vi "MattesImageRegistration.vi"(6 "Epsilon":dbl=0.01, 8 "error in (no error)":errorcluster, 9 "Starting Radius":dbl=10.0, 10 "Moving image in":T1=refnum, 11 "Fixed image in":T1=refnum) -> (0 "error out":errorcluster, 1 "False color alignment image":T1, 2 "Moving image out (duplicate)":T1, 3 "Fixed image out (duplicate)":T1, 4 "alignment quality":dbl=-0.39635115330155946, 5 "y translation":dbl=4.5810062720041405, 7 "x translation":dbl=-23.66339978067731)   [LabVIEW 2012]
uses:
  <vilib>/vision/Image Controls.llb/IMAQ Image.ctl
  <vilib>/vision/NI_Vision_Development_Module.lvlib
  C++/bin/Release/ImageReg.dll
panel:
  in  "maximum iteration":i32=200
  out "elapsed time (ms)":u32=741
  in  "Sampling Percentage":dbl=0.2
  out "# of iterations":dbl=100.0
  out "False color image":T1(plugin-control)
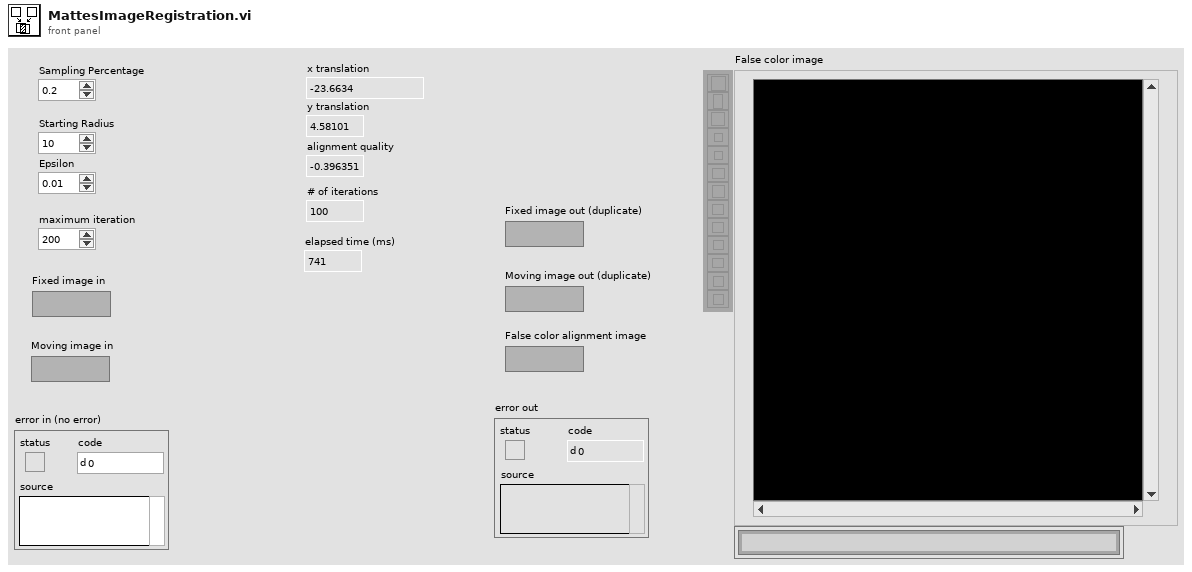
[diagram p1: front panel]
types:
  T1 = typedef "IMAQ Image.ctl" = refnum<image>
  T2 = typedef "Image Type" = u32
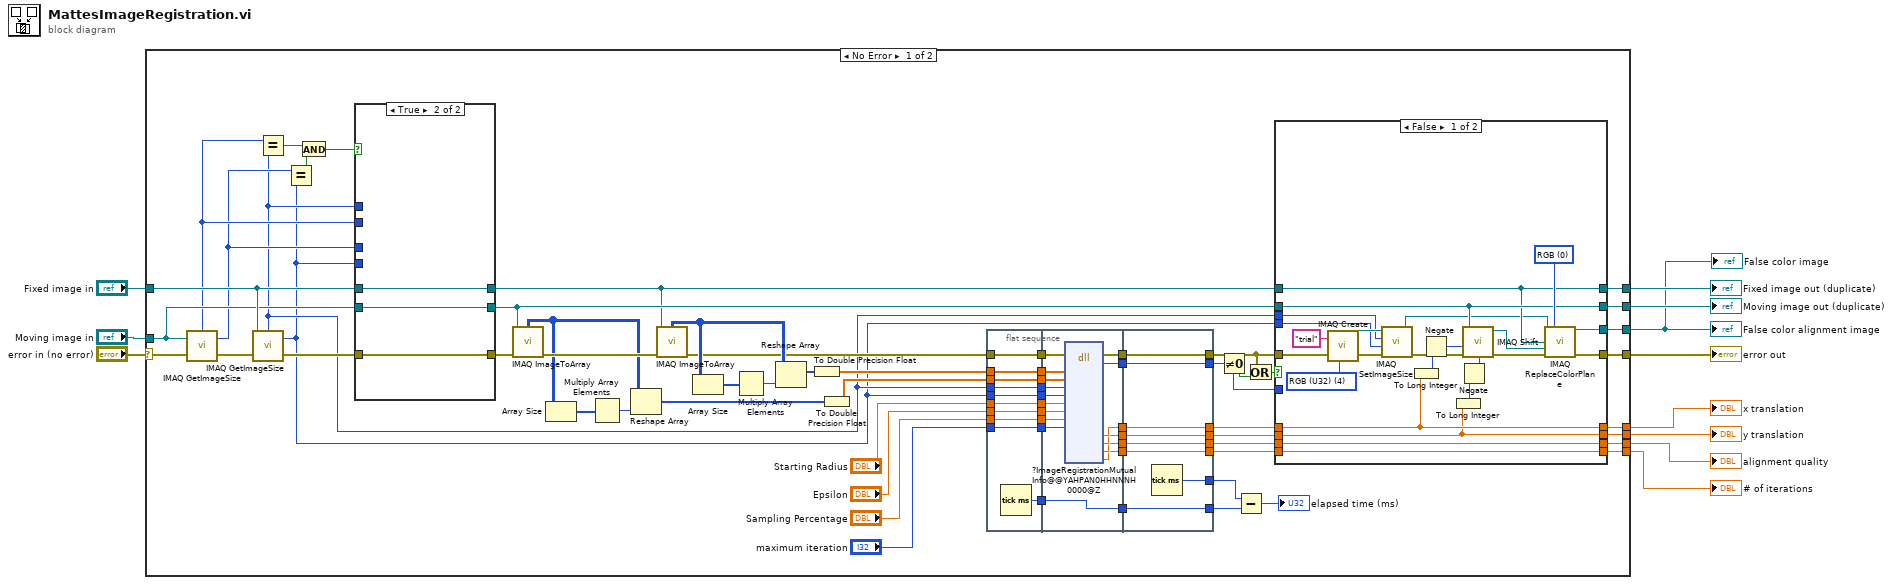
[diagram p0: block diagram]
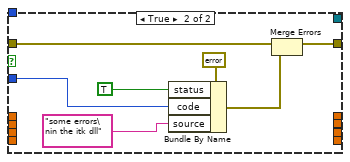
[diagram p2: hidden frame]
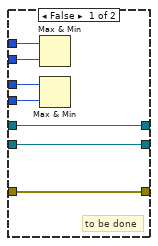
[diagram p3: hidden frame]
diagram:
  n1 = case shown="No Error" "error in (no error)" {
    selector: "error in (no error)" -> [w78 w154]
    tunnel: [w62 w154] -> w10
    tunnel: "Moving image in" -> [w72 _]
    tunnel: "Fixed image in" -> [w73 _]
    tunnel: [w53 _] -> w7
    tunnel: [w52 _] -> w6
    tunnel: [w51 _] -> w5
    tunnel: [w50 _] -> w2
    tunnel: [w49 _] -> w4
    tunnel: [w48 _] -> w3
    tunnel: [w47 _] -> w1
    frame No Error {
      n2 = call "IMAQ GetImageSize"("Image"=w72, "error in (no error)"=w78) -> ("Y Resolution"=w70:i32, "X Resolution"=w71:i32, "error out"=w77:errorcluster)  [unwired: 2 in]
      n3 = call "IMAQ GetImageSize"("Image"=w73, "error in (no error)"=w77) -> ("Y Resolution"=w41:i32, "X Resolution"=w42:i32, "error out"=w69:errorcluster)  [unwired: 2 in]
      n4 = Equal?(x=w71, y=w42) -> (x = y?=w75:bool)
      n5 = Equal?(x=w70, y=w41) -> (x = y?=w76:bool)
      n6 = And(x=w75, y=w76) -> (x .and. y?=w74:bool)
      n7 = case shown="True" w74 {
        tunnel: [w146 w153] -> w54
        tunnel: w73 -> [w146 w153]
        tunnel: [w145 w152] -> w61
        tunnel: w72 -> [w145 w152]
        tunnel: w42 -> [w150 _]
        tunnel: w71 -> [w149 _]
        tunnel: w70 -> [w148 _]
        tunnel: w41 -> [w147 _]
        tunnel: [w144 w151] -> w67
        tunnel: w69 -> [w144 w151]
        frame False {
          # "to be done"
          n8 = Max & Min(x=w150, y=w149) -> ()  [unwired: 2 out]
          n9 = Max & Min(x=w148, y=w147) -> ()  [unwired: 2 out]
        }
        frame True {
        }
      }
      n10 = call "IMAQ ImageToArray"("error in (no error)"=w67, "Image"=w61) -> ("error out"=w68:errorcluster, "Image Pixels (U8)"=w60:u8[][])  [unwired: 2 in, 3 out]
      n11 = Array Size(array=w60) -> (size(s)=w59:i32[])
      n12 = Multiply Array Elements(1:w59) -> (0:w58:i32)
      n13 = Reshape Array(w60, w58) -> (w65:u8[])
      n14 = call "IMAQ ImageToArray"("error in (no error)"=w68, "Image"=w54) -> ("error out"=w46:errorcluster, "Image Pixels (U8)"=w55:u8[][])  [unwired: 2 in, 3 out]
      n15 = Array Size(array=w55) -> (size(s)=w57:i32[])
      n16 = Multiply Array Elements(1:w57) -> (0:w56:i32)
      n17 = Reshape Array(w55, w56) -> (w66:u8[])
      n18 = To Double Precision Float(number=w66) -> (double precision float=w44:dbl[])
      n19 = To Double Precision Float(number=w65) -> (double precision float=w43:dbl[])
      n20 = flat-sequence {
        tunnel: "Sampling Percentage" -> [w81]
        tunnel: "Epsilon" -> [w82]
        tunnel: "Starting Radius" -> [w83]
        tunnel: w41 -> [w84]
        tunnel: w42 -> [w85]
        tunnel: w43 -> [w86]
        tunnel: w44 -> [w87]
        tunnel: w46 -> [w88]
        tunnel: [w88] -> w32
        tunnel: [w87] -> w31
        tunnel: [w86] -> w30
        tunnel: [w85] -> w29
        tunnel: [w84] -> w28
        tunnel: [w83] -> w27
        tunnel: [w82] -> w26
        tunnel: [w81] -> w25
        tunnel: [w80] -> w17
        tunnel: [w79] -> w13
        tunnel: "maximum iteration" -> [w79]
        tunnel: w32 -> [w104]
        tunnel: w31 -> [w102]
        tunnel: w30 -> [w101]
        tunnel: w29 -> [w100]
        tunnel: w28 -> [w99]
        tunnel: w27 -> [w98]
        tunnel: w26 -> [w97]
        tunnel: w25 -> [w96]
        tunnel: [w103] -> w24
        tunnel: [w95] -> w23
        tunnel: [w94] -> w22
        tunnel: [w93] -> w21
        tunnel: [w92] -> w20
        tunnel: [w91] -> w19
        tunnel: w17 -> [w90]
        tunnel: [w90] -> w16
        tunnel: w13 -> [w89]
        tunnel: [w107] -> w33
        tunnel: [w108] -> w34
        tunnel: [w109] -> w35
        tunnel: [w110] -> w36
        tunnel: [w111] -> w37
        tunnel: [w112] -> w45
        tunnel: w24 -> [w112]
        tunnel: w23 -> [w111]
        tunnel: w22 -> [w110]
        tunnel: w21 -> [w109]
        tunnel: w20 -> [w108]
        tunnel: w19 -> [w107]
        tunnel: [w106] -> w18
        tunnel: w16 -> [w105]
        tunnel: [w105] -> w15
        frame #0 {
          n21 = Tick Count (ms)() -> (millisecond timer value=w80:u32)
        }
        frame #1 {
          n22 = dll-call lib="D:/Moroder/dependencies/ImageReg/C++/bin/Release/ImageReg.dll" fn="?ImageRegistrationMutualInfo@@YAHPAN0HHNNNH0000@Z"(error in=w104, "fixed image"=w102, "moving image"=w101, "image width"=w100, "image height"=w99, "starting radius"=w98, "epsilon"=w97, "sampling percentage"=w96, "maximum iteration"=w89) -> (error out=w103:errorcluster, "error flag"=w91:i32, "x translation"=w95:dbl, "y translation"=w94:dbl, "quality"=w93:dbl, "number of iterations"=w92:dbl)  [unwired: 14 in, 1 out]
        }
        frame #2 {
          n23 = Tick Count (ms)() -> (millisecond timer value=w106:u32)
        }
      }
      n24 = Not Equal To 0?(x=w33) -> (x != 0?=w64:bool)
      n25 = Subtract(x=w18, y=w15) -> (x-y=→"elapsed time (ms)":u32)
      n26 = Or(x=w45, y=w64) -> (x .or. y?=w63:bool)
      n27 = case shown="False" w63 {
        tunnel: w45 -> [w132 w138]
        tunnel: w33 -> [_ w142]
        tunnel: [w133 w137] -> w62
        tunnel: w61 -> [w124 _]
        tunnel: w37 -> [w128 _]
        tunnel: w36 -> [w127 _]
        tunnel: w54 -> [w123 _]
        tunnel: [w128 _] -> w53
        tunnel: [w127 _] -> w52
        tunnel: [w126 _] -> w51
        tunnel: w35 -> [w126 _]
        tunnel: [w125 _] -> w50
        tunnel: [w124 _] -> w49
        tunnel: [w123 _] -> w48
        tunnel: [w117 _] -> w47
        tunnel: w34 -> [w117 _]
        tunnel: w42 -> [w114 _]
        tunnel: w41 -> [w113 _]
        frame False {
          w129 = u16 0 items=["RGB", "HSL", "HSV", "HSI"] ("Color Mode")
          w130 = T2 4 items=["Grayscale (U8)", "Grayscale (I16)", "Grayscale (SGL)", "Complex (CSG)", "RGB (U32)", "HSL (U32)", "RGB (U64)", "Grayscale (U16)"] ("Image Type")
          n28 = call "IMAQ Create"("Image Name"="trial", "Image Type"=w130, "error in (no error)"=w132) -> ("New Image"=w121:T1, "error out"=w116:errorcluster)  [unwired: 2 in]
          n29 = call "IMAQ SetImageSize"("error in (no error)"=w116, "Y Resolution"=w113, "X Resolution"=w114, "Image"=w121) -> ("error out"=w115:errorcluster, "Image Out"=w120:T1)  [unwired: 1 in]
          n30 = To Long Integer(number=w128) -> (32bit integer=w136:i32)
          n31 = Negate(x=w136) -> (-x=w119:i32)
          n32 = To Long Integer(number=w127) -> (32bit integer=w135:i32)
          n33 = Negate(x=w135) -> (-x=w118:i32)
          n34 = call "IMAQ Shift"("YOffset"=w118, "error in (no error)"=w115, "XOffset"=w119, "Image Src"=w124) -> ("error out"=w134:errorcluster, "Image Dst Out"=w122:T1)  [unwired: 6 in]
          n35 = call "IMAQ ReplaceColorPlane"("Image Src"=w120, "Color Mode"=w129, "Red or Hue Plane"=w123, "Green or Sat Plane"=w122, "error in (no error)"=w134) -> ("Image Dst Out"=w125:T1, "error out"=w133:errorcluster)  [unwired: 9 in]
        }
        frame True {
          n36 = Bundle By Name(cluster=errorcluster {"status"=FALSE, "code"=0, "source"=""} ("error in"), "status"=TRUE, "code"=w142, "source"="some errors\nin the itk dll") -> (w139:errorcluster)
          n37 = Merge Errors(w138, w139) -> (w137:errorcluster)
        }
      }
    }
    frame Error {
    }
  }
  "error out" <- w10
  "x translation" <- w7
  "y translation" <- w6
  "alignment quality" <- w5
  "Fixed image out (duplicate)" <- w3
  "Moving image out (duplicate)" <- w4
  "False color alignment image" <- w2
  "False color image" <- w2
  "# of iterations" <- w1
